vi "Pre-Build Action.vi"(6 "Top Level/Always Included VIs":path[](array[path]), 7 "Main Destination Path":path, 9 "Target Name":string, 10 "Build Specification Name":string, 11 "Project Path":path) -> (0 "error out":errorcluster)   [LabVIEW 2020]
panel:
  out "Revision number":i32
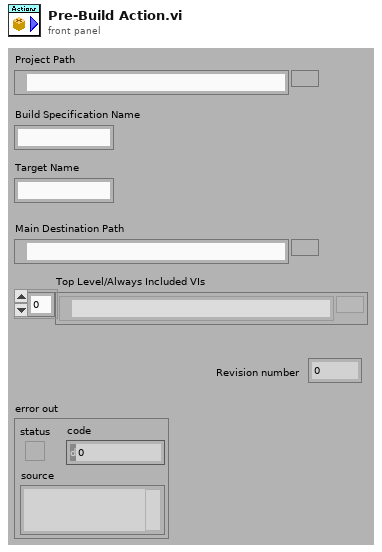
[diagram p1: front panel]
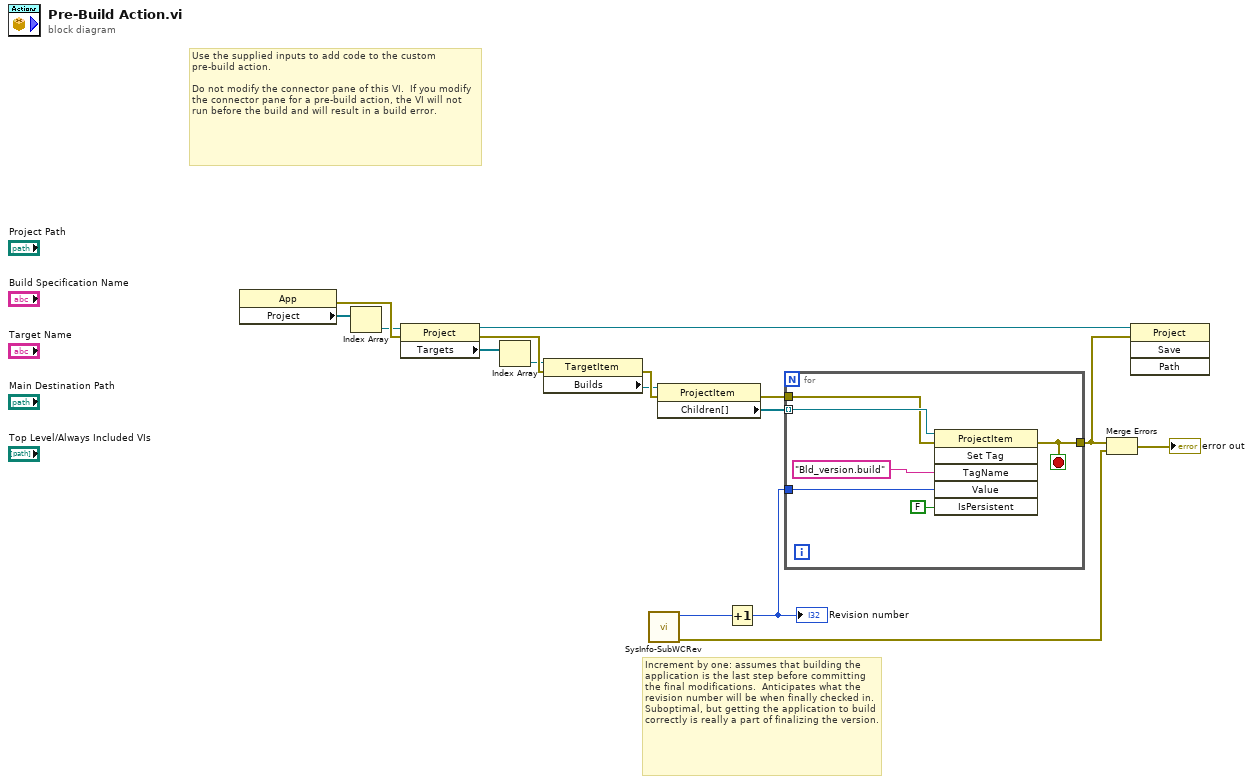
[diagram p0: block diagram]
diagram:
  # "Increment by one: assumes that building the application is the last step before committing the final modifications.  Anticipates what the revision number will be when finally checked in. Suboptimal, but getting the application to build correctly is really a part of finalizing the version."
  # "Use the supplied inputs to add code to the custom pre-build action.\n\nDo not modify the connector pane of this VI.  If you modify the connector pane for a pre-build action, the VI will not run before the build and will result in a build error."
  n1 = property class="App"() -> (error out=w16:errorcluster, "Project"=w13:refnum<vi>[])  [unwired: 2 in, 1 out]
  n2 = Index Array(array=w13) -> (element=w12:refnum<vi>)  [unwired: 1 in]
  n3 = property class="Project"(reference=w12, error in=w16) -> (reference out=w3:refnum<vi>, error out=w15:errorcluster, "Targets"=w11:refnum<vi>[])
  n4 = Index Array(array=w11) -> (element=w10:refnum<vi>)  [unwired: 1 in]
  n5 = property class="TargetItem"(reference=w10, error in=w15) -> (error out=w14:errorcluster, "Builds"=w9:refnum<vi>)  [unwired: 1 out]
  n6 = call "SysInfo-SubWCRev.vi"() -> ("error out"=w5:errorcluster, "Revision"=w6:i32)  [unwired: 9 in, 1 out]
  n7 = property class="ProjectItem"(reference=w9, error in=w14) -> (error out=w8:errorcluster, "Children[]"=w7:refnum<vi>[])  [unwired: 1 out]
  n8 = Increment(x=w6) -> (x+1=w1:i32)
  "Revision number" <- w1
  n9 = for {
    tunnel: w8 -> [w19]
    tunnel: w7 -> [w20] mode=indexing
    tunnel: [w18] -> w4
    tunnel: w1 -> [w17]
    stop <- w18 stop-if-true
    n10 = invoke class="ProjectItem" method="Set Tag"(reference=w20, error in=w19, "TagName"="Bld_version.build", "Value"=w17, "IsPersistent"=FALSE ("Is Persistent")) -> (error out=w18:errorcluster)  [unwired: 1 in, 5 out]
  }
  n11 = Merge Errors(w4, w5) -> (→"error out":errorcluster)
  n12 = invoke class="Project" method="Save"(reference=w3, error in=w4) -> ()  [unwired: 2 in, 4 out]
